vi "Get Setpoint.vi"(0 "Session Handle":T1, 11 "error in (no error)":errorcluster) -> (4 "Session Handle Out":T1, 6 "Set Point":dbl, 15 "error out":errorcluster)   [LabVIEW 2015, in "Peltier.lvclass"]
uses:
  Peltier.lvclass
  Typedefs/Session Handle.ctl
  Gas/Gas.lvclass
panel:
  out "Success?":bool
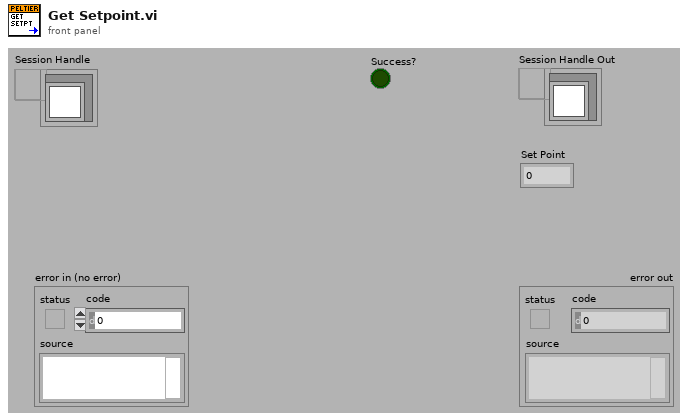
[diagram p1: front panel]
types:
  T1 = typedef "Peltier.lvclass/Session Handle.ctl" = refnum<data-value>
  T2 = typedef "XNET Frame CAN.ctl" = cluster{"timestamp":timestamp, "payload":u8[], "identifier":u32, "type":T3, "extended?":bool, "echo?":bool}
  T3 = typedef "XNET Frame Type CAN.ctl" = u8
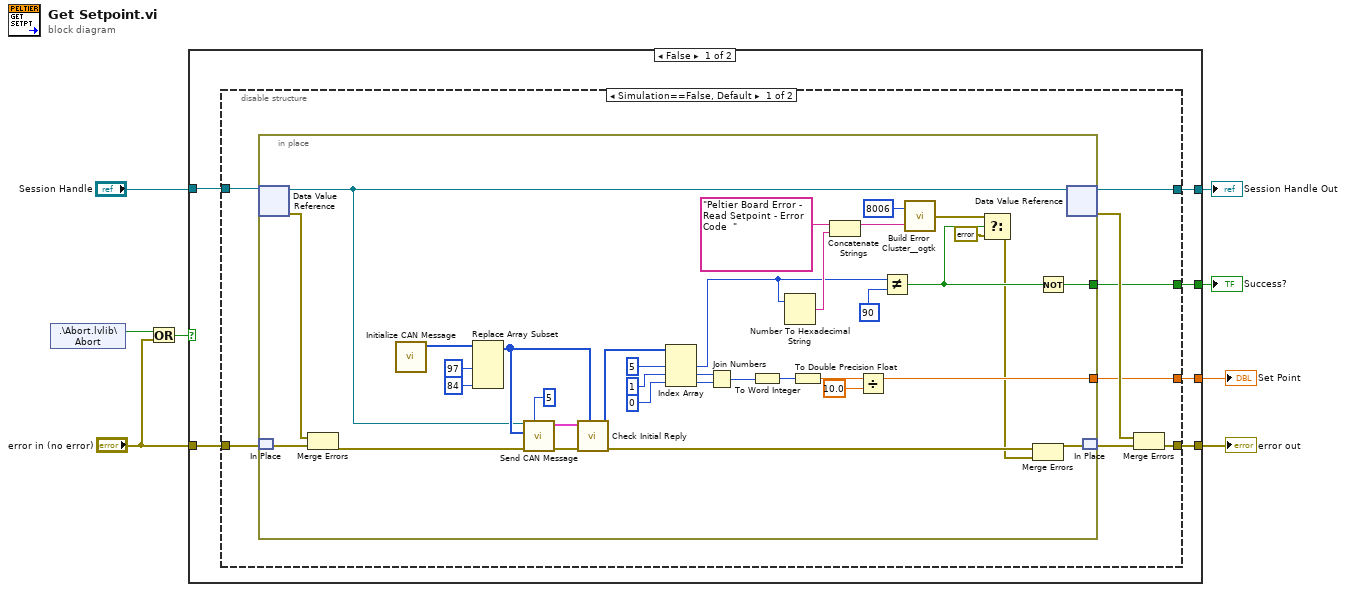
[diagram p0: block diagram]
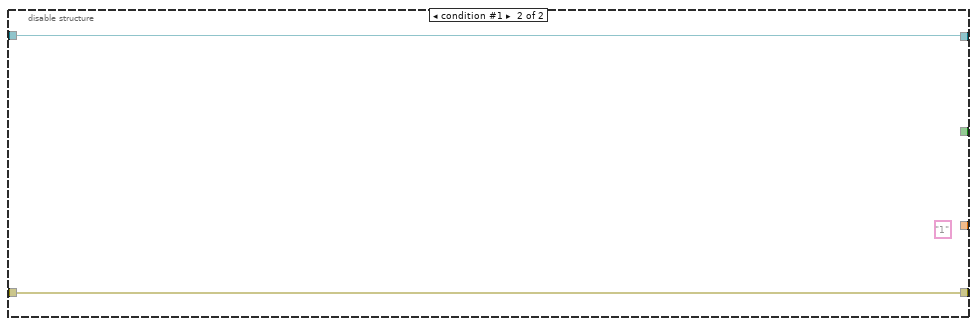
[diagram p2: hidden frame]
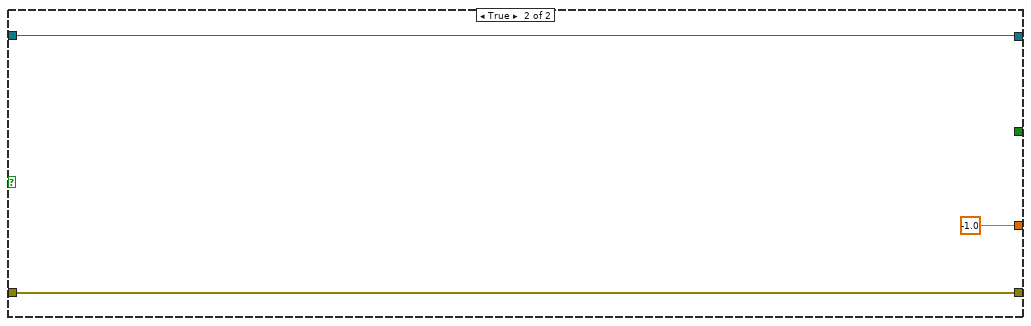
[diagram p3: hidden frame]
diagram:
  n1 = shared-variable ".\\Abort.lvlib\\Abort"() -> (w7:bool)  [unwired: 1 in, 1 out]
  n2 = Or(x=w7, y="error in (no error)") -> (x .or. y?=w5:bool)
  n3 = case shown="False" w5 {
    tunnel: [w14 w62] -> w1
    tunnel: [w13 w61] -> w8
    tunnel: "Session Handle" -> [w12 w62]
    tunnel: "error in (no error)" -> [w11 w61]
    tunnel: [w10 -1.0] -> w4
    tunnel: [w9 _] -> w3
    frame False {
      n4 = disable-structure shown="Simulation==False, Default" {
        disable-tunnel: [w22 w59] -> w14
        disable-tunnel: [w19 w58] -> w13
        disable-tunnel: w12 -> [w18 w59]
        disable-tunnel: w11 -> [w17 w58]
        disable-tunnel: [w16 _] -> w10
        disable-tunnel: [w15 _] -> w9
        frame condition #0 (active) {
          n5 = in-place {
            in-place-border: [w27] -> w16
            in-place-border: [w39] -> w15
            n6 = in-place-dvr #1(w18) -> (w48:refnum<class "Peltier.lvclass">, w53:errorcluster)
            n7 = in-place-match #2(w17) -> (w52:errorcluster)
            n8 = Merge Errors(w53, w52) -> (w47:errorcluster)
            n9 = call "Initialize CAN Message.vi"() -> ("Initial Payload"=w55:u8[])  [unwired: 11 in]
            n10 = Replace Array Subset(array=w55, new element #1=u8 97 ("new element/subarray"), new element #2=u8 84 ("new element/subarray")) -> (w51:u8[])  [unwired: 2 in]
            n11 = call "Send CAN Message.vi"("Number of Retries"=5, "error in (no error)"=w47, "payload"=w51, "Peltier In"=w48) -> ("error out"=w25:errorcluster, "Reply"=w49:T2[])  [unwired: 5 in, 1 out]
            n12 = call "Check Initial Reply.vi"("Write Message"=w51, "error in (no error)"=w25, "Reply"=w49) -> ("error out"=w24:errorcluster, "Data Packet"=w54:u8[])  [unwired: 5 in, 2 out]
            n13 = Index Array(array=w54, index #1=5 ("index"), index #2=1 ("index"), index #3=0 ("index")) -> (element #1=w40:u8, element #2=w35:u8, element #3=w34:u8)
            n14 = Join Numbers(hi=w35, lo=w34) -> ((hi.lo)=w33:u16)
            n15 = To Word Integer(number=w33) -> (16bit integer=w36:i16)
            n16 = Number To Hexadecimal String(2:w40) -> (0:w44:string)  [unwired: 1 in]
            n17 = To Double Precision Float(number=w36) -> (double precision float=w29:dbl)
            n18 = Concatenate Strings("Peltier Board Error -  Read Setpoint - Error Code  " ("string"), w44) -> (w43:string)
            n19 = Divide(x=w29, y=10.0) -> (x/y=w27:dbl)
            n20 = Not Equal?(x=w40, y=u8 90 ("new element/subarray")) -> (x != y?=w30:bool)
            n21 = call <userlib>:"Build Error Cluster__ogtk.vi"("String to Prepend to source (\"\")"=w43, "code"=8006) -> ("error out"=w32:errorcluster)
            n22 = Select(t=w32, s=w30, f=errorcluster {"status"=FALSE, "code"=0, "source"=""}) -> (s? t:f=w23:errorcluster)
            n23 = Merge Errors(w24, w23) -> (w56:errorcluster)
            n24 = Not(x=w30) -> (.not. x?=w39:bool)
            n25 = in-place-dvr #1(w48) -> (w22:T1, w20:errorcluster)
            n26 = in-place-match #2(w56) -> (w21:errorcluster)
          }
          n27 = Merge Errors(w20, w21) -> (w19:errorcluster)
        }
        frame condition #1 {
          (unwired) "1"
        }
      }
    }
    frame True {
    }
  }
  "error out" <- w8
  "Set Point" <- w4
  "Success?" <- w3
  "Session Handle Out" <- w1
